vi "Temp_2.0.vi"() -> ()   [LabVIEW 2020]
uses:
  <vilib>/Instr/_visa.llb/VISA Configure Serial Port (Instr).vi
panel:
  in  "stop":bool
  out "number":dbl
  in  "VISA resource name":refnum<visa-resource-name>
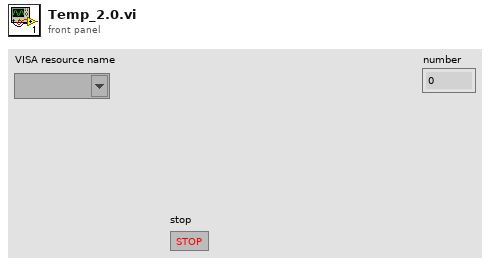
[diagram p1: front panel]
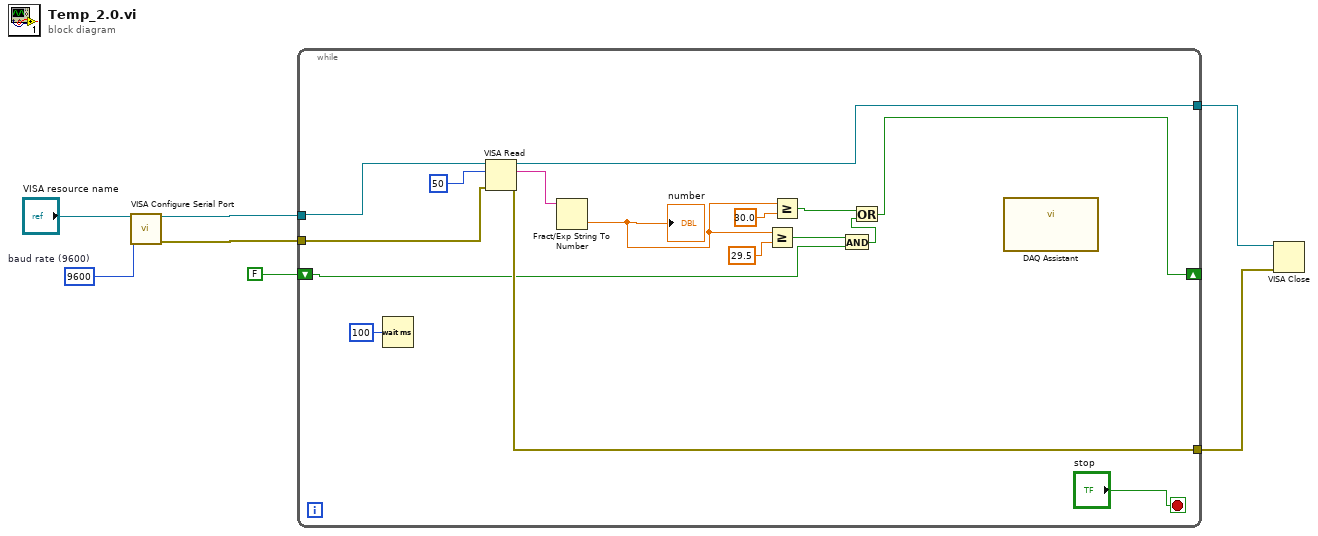
[diagram p0: block diagram]
diagram:
  w6 = u32 9600  # baud rate (9600)
  n1 = call-poly "VISA Configure Serial Port"("VISA resource name"="VISA resource name", "baud rate (9600)"=w6) -> ("VISA resource name out"=w5:refnum<visa-resource-name>, "error out"=w4:errorcluster)  [unwired: 12 in]
  n2 = while {
    tunnel: w5 -> [w22]
    tunnel: w4 -> [w21]
    tunnel: [w18] -> w3
    tunnel: [w17] -> w2
    shift-right: [w8] -> _
    shift-left: FALSE -> [w10]
    stop <- "stop" stop-if-true
    n3 = Wait (ms)(milliseconds to wait=u32 100) -> ()  [unwired: 1 out]
    n4 = VISA Read(VISA resource name=w22, byte count=u32 50, error in (no error)=w21) -> (VISA resource name out=w18:refnum<visa-resource-name>, read buffer=w19:string, error out=w17:errorcluster)  [unwired: 1 out]
    n5 = Fract/Exp String To Number(string=w19) -> (number=w14:dbl)  [unwired: 3 in, 1 out]
    "number" <- w14
    n6 = Greater Or Equal?(x=w14, y=29.5) -> (x >= y?=w12:bool)
    n7 = Greater Or Equal?(x=w14, y=30.0) -> (x >= y?=w11:bool)
    n8 = And(x=w12, y=w10) -> (x .and. y?=w9:bool)
    n9 = Or(x=w11, y=w9) -> (x .or. y?=w8:bool)
    n10 = call "DAQ Assistant"() -> ()  [unwired: 12 in]
  }
  n11 = VISA Close(VISA resource name=w3, error in (no error)=w2) -> ()  [unwired: 1 out]
